vi "SaveCUTReport.vi"(6 "TemplateName":string="CUT Uncertainties.xltx", 8 "error in (no error)":errorcluster, 10 "MeanStdSlope":dbl[][](array[numeric]), 11 "Results Table":string[][](table)) -> (0 "error out":errorcluster)   [LabVIEW 2014]
uses:
  Excel(ActiveX)/enumOpenOrCreate.ctl
  typedefs/ePathsAction.ctl
  Excel(ActiveX)/Excel(ActiveX).lvlib
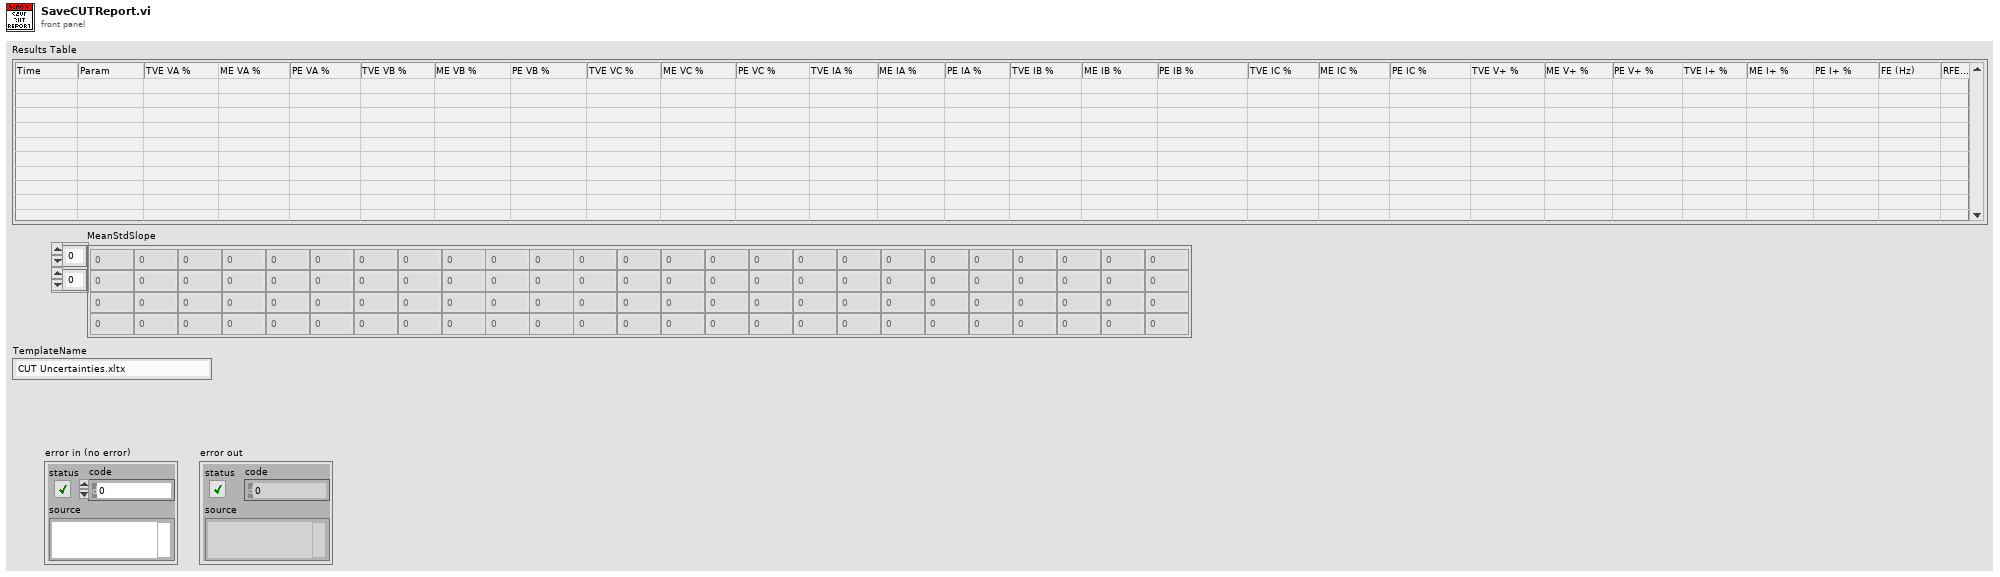
[diagram p1: front panel]
types:
  T1 = typedef "ePathsAction.ctl" = enum16{"Set", "Get", "Load", "Save", "Default", "Exit"}
  T2 = typedef "Excel(ActiveX).lvlib/enumOpenOrCreate.ctl" = enum16{"open", "open or create", "create from template"}
  T3 = typedef "Excel(ActiveX).lvlib/ExcelActiveX.ctl" = cluster{"Excel._Application":refnum<k7>, "Application open at start":bool, "Excel._Worksheet":refnum<k7>, "Workbook open at start":bool, "Excel._Workbook":refnum<k7>, "Workbook Path":path, "Worksheet Name":string, "Row":u32, "Col":u32, "Cell":string, "Workbook Name":string}
  T4 = typedef "Paths.ctl" = cluster{"BasePath":path, "CutPath":path, "LastCutPath":path, "CCSPath":path, "LastCCSPath":path, "ResultsPath":path}
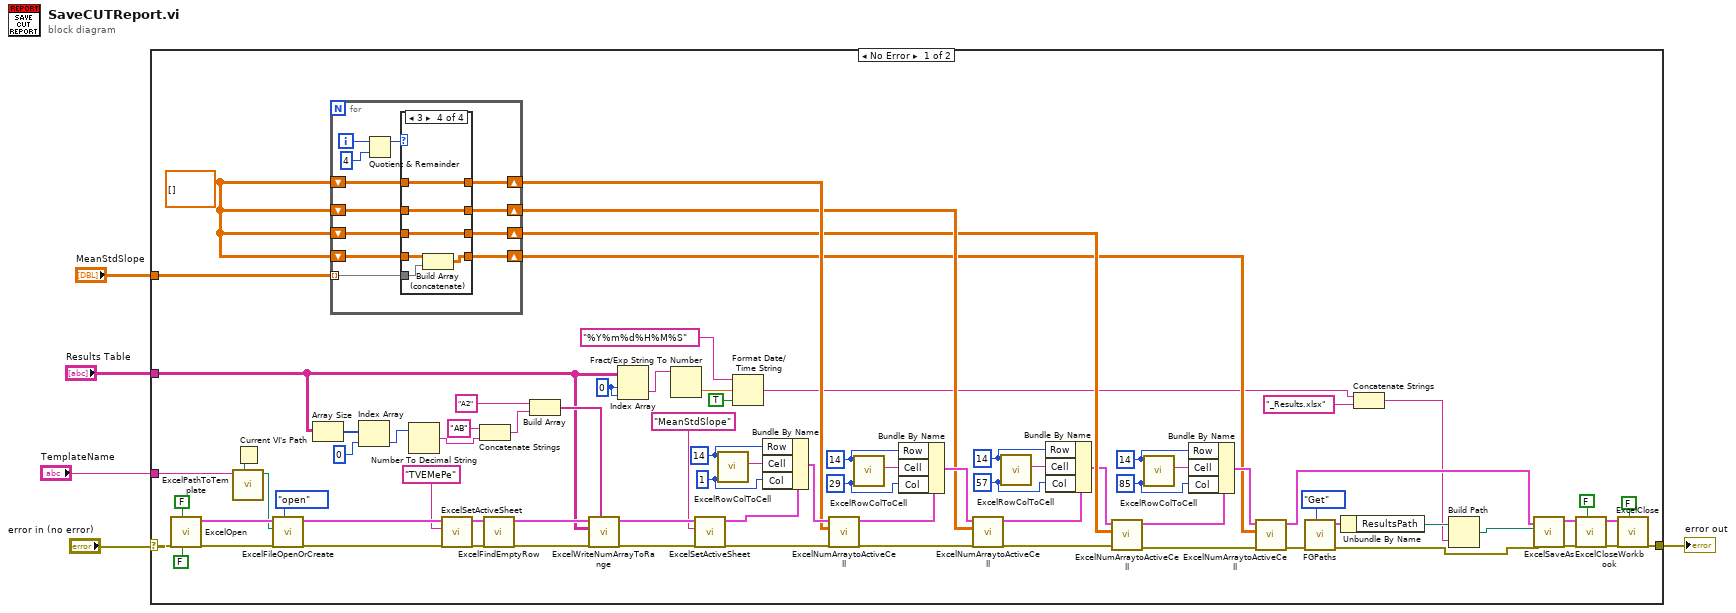
[diagram p0: block diagram]
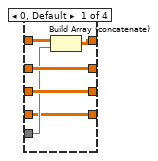
[diagram p2: hidden frame]
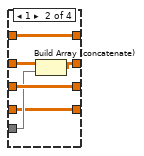
[diagram p3: hidden frame]
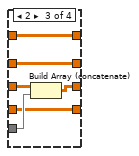
[diagram p4: hidden frame]
diagram:
  n1 = case shown="No Error" "error in (no error)" {
    selector: "error in (no error)" -> [w85 w122]
    tunnel: [w84 w122] -> w4
    tunnel: "Results Table" -> [w16 _]
    tunnel: "MeanStdSlope" -> [w83 _]
    tunnel: "TemplateName" -> [w22 _]
    frame No Error {
      w15 = 0 ("index (row)")
      w42 = u32 85 ("col")
      w40 = u32 14 ("row")
      w48 = u32 57 ("col")
      w50 = u32 14 ("row")
      w57 = u32 29 ("col")
      w55 = u32 14 ("row")
      w61 = u32 1 ("col")
      w63 = u32 14 ("row")
      w43 = dbl[][] []
      n2 = call "ExcelOpen.vi"("Run Minimized (f)"=FALSE, "Excel visible? (t)"=FALSE, "error in (no error)"=w85) -> ("error out"=w79:errorcluster, "ExcelActiveX"=w78:T3)  [unwired: 7 in]
      n3 = Current VI's Path() -> (path=w82:path)
      n4 = call "ExcelPathToTemplate.vi"("PathToCallingVI"=w82, "TemplateName"=w22) -> ("template"=w76:path)  [unwired: 8 in, 1 out]
      n5 = call "ExcelFileOpenOrCreate.vi"("Open or Create"=enumOpenOrCreate."open", "error in (no error)"=w79, "Excel file name and path"=w76, "ExcelActiveX in"=w78) -> ("error out"=w69:errorcluster, "ExcelActiveX out"=w68:T3)  [unwired: 6 in]
      n6 = Array Size(array=w16) -> (size(s)=w30:i32[])
      n7 = for {
        tunnel: w83 -> [w94] mode=indexing
        shift-right: [w92] -> w58
        shift-left: w43 -> [w93]
        shift-right: [w90] -> w51
        shift-left: w43 -> [w91]
        shift-right: [w88] -> w46
        shift-left: w43 -> [w89]
        shift-right: [w86] -> w36
        shift-left: w43 -> [w87]
        i -> [w97]
        n8 = Quotient & Remainder(x=w97, y=4) -> (x-y*floor(x/y)=w95:i32)  [unwired: 1 out]
        n9 = case shown="3" w95 {
          tunnel: w94 -> [w99 w106 w111 w119]
          tunnel: w93 -> [w101 w105 w115 w121]
          tunnel: [w100 w105 w115 w121] -> w92
          tunnel: [w102 w107 w114 w120] -> w90
          tunnel: w91 -> [w102 w108 w114 w120]
          tunnel: w89 -> [w103 w109 w113 w118]
          tunnel: [w103 w109 w112 w118] -> w88
          tunnel: w87 -> [w98 w104 w110 w117]
          tunnel: [w98 w104 w110 w116] -> w86
          frame 0, Default {
            n10 = Build Array (concatenate)(w101, w99) -> (w100:dbl[][])
          }
          frame 1 {
            n11 = Build Array (concatenate)(w108, w106) -> (w107:dbl[][])
          }
          frame 2 {
            n12 = Build Array (concatenate)(w113, w111) -> (w112:dbl[][])
          }
          frame 3 {
            n13 = Build Array (concatenate)(w117, w119) -> (w116:dbl[][])
          }
        }
      }
      n14 = Index Array(array=w30, index=0) -> (element=w28:i32)
      n15 = Number To Decimal String(number=w28) -> (decimal integer string=w26:string)  [unwired: 1 in]
      n16 = call "ExcelSetActiveSheet.vi"("error in (no error)"=w69, "Sheet Name"="TVEMePe", "ExcelActiveX in"=w68) -> ("error out"=w34:errorcluster, "ExcelActiveX  out"=w33:T3)  [unwired: 7 in]
      n17 = Concatenate Strings("AB", w26) -> (w24:string)
      n18 = call "ExcelFindEmptyRow.vi"("error in (no error)"=w34, "ExcelActiveX"=w33) -> ("error out"=w32:errorcluster, "ExcelActiveX"=w31:T3)  [unwired: 8 in]
      n19 = Build Array("A2", w24) -> (w23:string[])
      n20 = call "ExcelWriteNumArrayToRange.vi"("Range"=w23, "error in (no error)"=w32, "StringArray"=w16, "ExcelActiveX"=w31) -> ("error out"=w66:errorcluster, "ExcelActiveX"=w67:T3)  [unwired: 6 in]
      n21 = Index Array(array=w16, index (row)=w15, index (col)=w15) -> (element=w14:string)
      n22 = Fract/Exp String To Number(string=w14) -> (number=w13:dbl)  [unwired: 3 in, 1 out]
      n23 = call "ExcelSetActiveSheet.vi"("error in (no error)"=w66, "Sheet Name"="MeanStdSlope", "ExcelActiveX in"=w67) -> ("error out"=w60:errorcluster, "ExcelActiveX  out"=w64:T3)  [unwired: 7 in]
      n24 = call "ExcelRowColToCell.vi"("col"=w61, "row"=w63) -> ("cell"=w62:string)  [unwired: 9 in]
      n25 = Format Date/Time String(time format string (%c)="%Y%m%d%H%M%S", seconds (now)=w13, UTC format=TRUE) -> (date/time string=w8:string)
      n26 = Bundle By Name(cluster=w64, "Row"=w63, "Cell"=w62, "Col"=w61) -> (w59:T3)
      n27 = call "ExcelNumArraytoActiveCell.vi"("error in (no error)"=w60, "Num Array"=w58, "ExcelActiveX"=w59) -> ("error out"=w53:errorcluster, "ExcelActiveX"=w54:T3)  [unwired: 7 in]
      n28 = call "ExcelRowColToCell.vi"("col"=w57, "row"=w55) -> ("cell"=w56:string)  [unwired: 9 in]
      n29 = Bundle By Name(cluster=w54, "Row"=w55, "Cell"=w56, "Col"=w57) -> (w52:T3)
      n30 = call "ExcelNumArraytoActiveCell.vi"("error in (no error)"=w53, "Num Array"=w51, "ExcelActiveX"=w52) -> ("error out"=w44:errorcluster, "ExcelActiveX"=w47:T3)  [unwired: 7 in]
      n31 = call "ExcelRowColToCell.vi"("col"=w48, "row"=w50) -> ("cell"=w49:string)  [unwired: 9 in]
      n32 = Bundle By Name(cluster=w47, "Row"=w50, "Cell"=w49, "Col"=w48) -> (w45:T3)
      n33 = call "ExcelNumArraytoActiveCell.vi"("error in (no error)"=w44, "Num Array"=w46, "ExcelActiveX"=w45) -> ("error out"=w39:errorcluster, "ExcelActiveX"=w38:T3)  [unwired: 7 in]
      n34 = call "ExcelRowColToCell.vi"("col"=w42, "row"=w40) -> ("cell"=w41:string)  [unwired: 9 in]
      n35 = Bundle By Name(cluster=w38, "Row"=w40, "Cell"=w41, "Col"=w42) -> (w37:T3)
      n36 = call "ExcelNumArraytoActiveCell.vi"("error in (no error)"=w39, "Num Array"=w36, "ExcelActiveX"=w37) -> ("error out"=w21:errorcluster, "ExcelActiveX"=w19:T3)  [unwired: 7 in]
      n37 = call "FGPaths.vi"("ePathsAction"=ePathsAction."Get", "error in (no error)"=w21) -> ("error out"=w20:errorcluster, "PathsOut"=w17:T4)  [unwired: 8 in]
      n38 = Unbundle By Name(w17) -> ("ResultsPath"=w10:path)
      n39 = Concatenate Strings(w8, "_Results.xlsx") -> (w7:string)
      n40 = Build Path(base path=w10, name or relative path=w7) -> (appended path=w6:path)
      n41 = call "ExcelSaveAs.vi"("error in (no error)"=w20, "Path"=w6, "ExcelActiveX"=w19) -> ("error out"=w72:errorcluster, "ExcelActiveX"=w71:T3)  [unwired: 7 in]
      n42 = call "ExcelCloseWorkbook.vi"("Save"=FALSE, "error in (no error)"=w72, "ExcelActiveX"=w71) -> ("error out"=w74:errorcluster, "ExcelActiveX"=w70:T3)  [unwired: 7 in]
      n43 = call "ExcelClose.vi"("Leave Open (f)"=FALSE, "error in (no error)"=w74, "ExcelActiveX in"=w70) -> ("error out"=w84:errorcluster)  [unwired: 7 in, 1 out]
    }
    frame Error {
    }
  }
  "error out" <- w4
